vi "Read.vi"(8 "error in (no error)":errorcluster, 11 "Keithley 2000 in":refnum<class "Keithley 2000.lvclass">) -> (0 "error out":errorcluster, 1 "Unit":string, 2 "Measure":dbl, 3 "Keithley 2000 out":refnum<class "Keithley 2000.lvclass">, 4 "Channel":i32)   [LabVIEW 2020, in "Keithley 2000.lvclass"]
uses:
  Keithley 2000.lvclass
  C:/Sandbox/Git_Sandbox/WiSpry Test Framework source code (LV20)/WiSpry Test Framework/Instruments/Instrument.lvclass
  Instrument.lvclass/Instrument.ctl
  Instrument.lvclass
  <instrlib>/Keithley 2000/Keithley 2000.lvlib
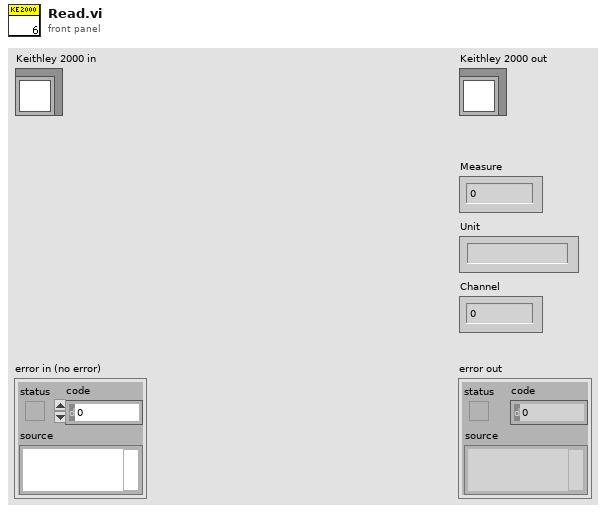
[diagram p1: front panel]
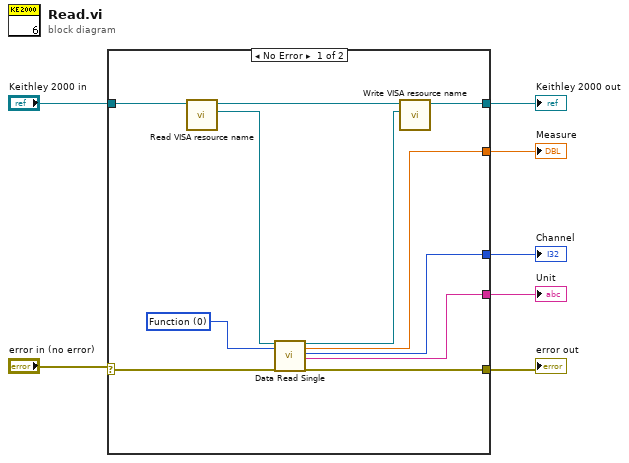
[diagram p0: block diagram]
diagram:
  n1 = case shown="No Error" "error in (no error)" {
    selector: "error in (no error)" -> [w15 w20]
    tunnel: [w12 w20] -> w6
    tunnel: "Keithley 2000 in" -> [w18 w19]
    tunnel: [w16 w19] -> w5
    tunnel: [w11 _] -> w3
    tunnel: [w10 _] -> w2
    tunnel: [w9 _] -> w1
    frame No Error {
      w8 = u16 0 items=["Function", "Calculation 1", "Calculation 2", "Calculation 3"] ("Source (0: Function)")
      n2 = call "Read VISA resource name.vi"("Instrument in"=w18) -> ("VISA resource name"=w14:refnum<visa-resource-name>, "Instrument out"=w17:refnum<class "Keithley 2000.lvclass">)  [unwired: 9 in]
      n3 = call <instrlib>:"Data Read Single.vi"("VISA resource name"=w14, "Source (0: Function)"=w8, "error in (no error)"=w15) -> ("VISA resource name out"=w13:refnum<visa-resource-name>, "Measurement"=w11:dbl, "Channel"=w10:i32, "Units"=w9:string, "error out"=w12:errorcluster)  [unwired: 12 in]
      n4 = call "Write VISA resource name.vi"("VISA resource name"=w13, "Instrument in"=w17) -> ("Instrument out"=w16:refnum<class "Keithley 2000.lvclass">)  [unwired: 9 in]
    }
    frame Error {
    }
  }
  "error out" <- w6
  "Keithley 2000 out" <- w5
  "Measure" <- w3
  "Unit" <- w1
  "Channel" <- w2
